vi "Kinesis - BPC301 - Connect.vi"() -> ()   [LabVIEW 2012]
uses:
  U:/Kinesis LabVIEW Website Examples/Thorlabs.MotionControl.Controls.dll
  Thorlabs.MotionControl.Controls.dll
panel:
  in  "?":bool
  in  "SerialNumber":string
  in  "BenchtopPiezoControl":refnum<k24>(container)
  # "Notes:"
  # "- Ensure that the appropriate .DLLs are copied into your Project Folder. Check that the correct bit type are used depending on your version of LabVIEW\ni.e. 32-bit or 64-bit.\n\n\n\n\n\n\n\n\n\n\n\n\n\n\n- Open the example VI through the LabVIEW Project Explorer to correctly load the User Interface from Thorlabs.MotionControl.Controls.dll."
  # "Thorlabs Hardware: BPC301 - 1-Channel Benchtop Piezo Controller\nhttps://www.thorlabs.com/newgrouppage9.cfm?objectgroup_id=1912&pn=BPC301\n\nDescription: This VI shows you how to initialize communication with and then disconnect the BPC301 controller.\n\nInstructions: \n1) Connect your BPC301 device to your PC & power the device.\nFor full device setup, the device product manual can be found on our website here. - https://www.thorlabs.com/thorproduct.cfm?partnumber=BPC301\n2) Enter the device serial number below.\n3) Click 'Run' in the LabVIEW Toolbar.\n4) To End the progam, click the 'STOP' button."
  # "Example Image of .NET Controller - VI opened via Project Explorer/ not opened via Project Explorer"
  # "VI Not Opened via Project Explorer"
  # "VI Opened via Project Explorer"
  # "- To explore the range of methods available, please visit the .NET API, included with your Kinesis software.\n\n- For tips on building your own VIs with Thorlabs Motion Control Hardware, please see our LabVIEW Guide here.\nhttps://www.thorlabs.com/newgrouppage9.cfm?objectgroup_id=10285"
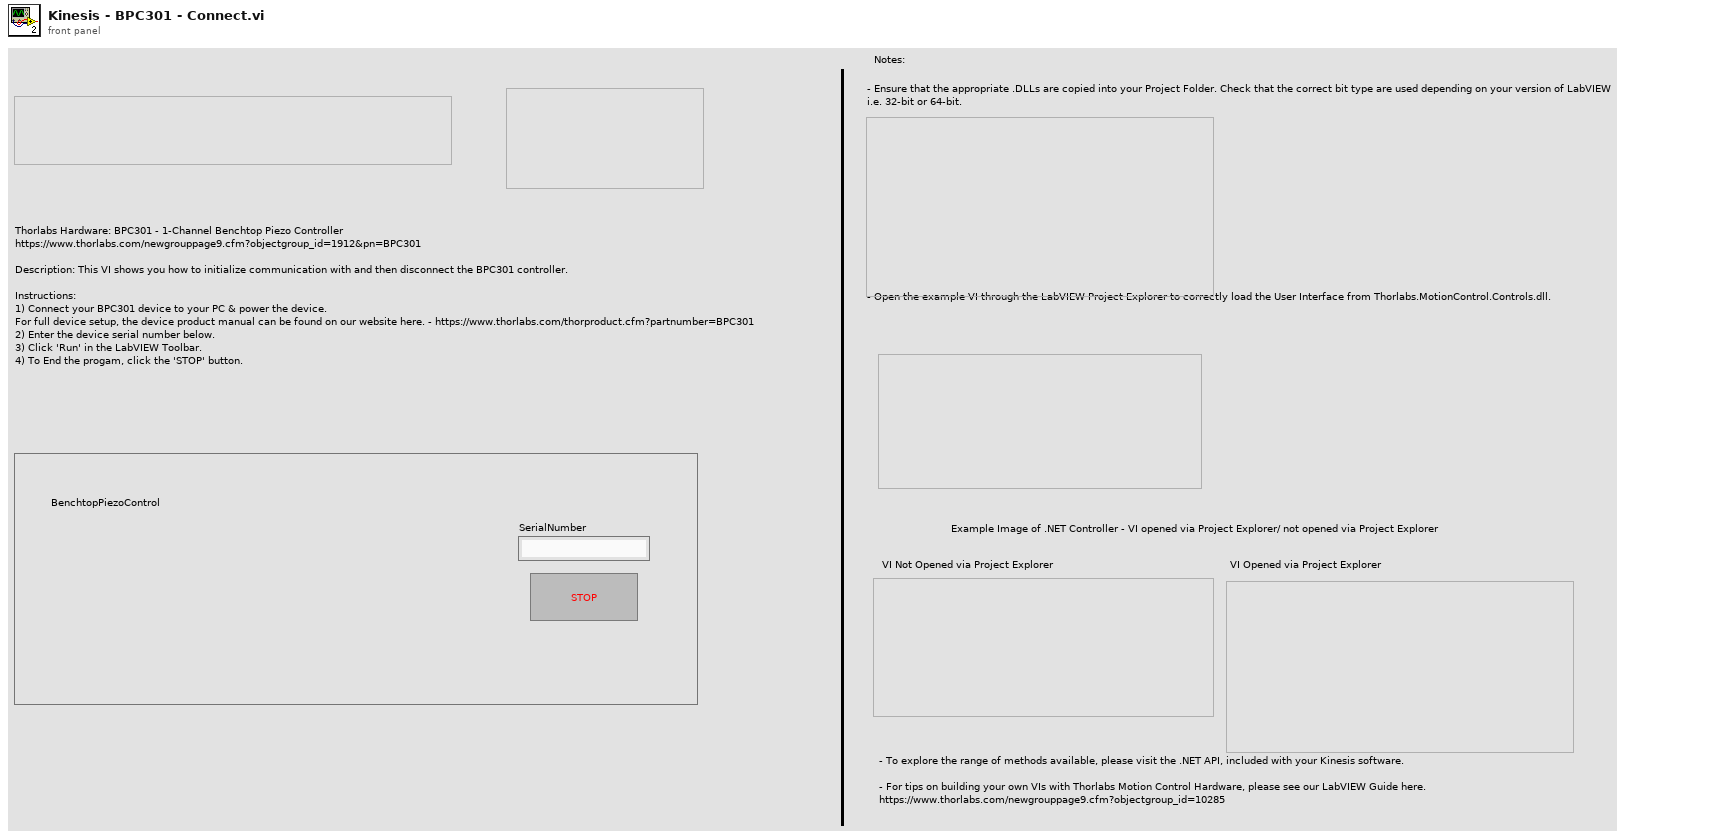
[diagram p1: front panel]
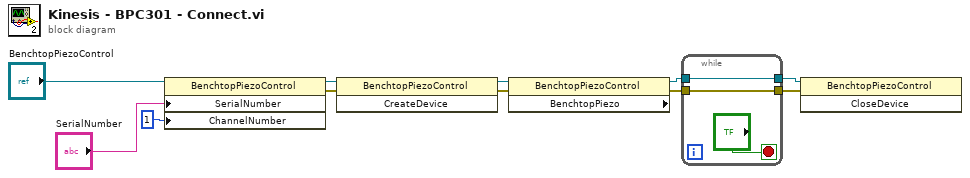
[diagram p0: block diagram]
diagram:
  n1 = property class="BenchtopPiezoControl"(reference="BenchtopPiezoControl", "SerialNumber"="SerialNumber", "ChannelNumber"=1) -> (reference out=w8:refnum<k24>, error out=w6:errorcluster)  [unwired: 1 in]
  n2 = invoke class="BenchtopPiezoControl" method="CreateDevice"(reference=w8, error in=w6) -> (reference out=w7:refnum<k24>, error out=w5:errorcluster)  [unwired: 1 in, 1 out]
  n3 = property class="BenchtopPiezoControl" props=["BenchtopPiezo"](reference=w7, error in=w5) -> (reference out=w1:refnum<k24>, error out=w3:errorcluster)  [unwired: 1 out]
  n4 = while {
    tunnel: [w14] -> w4
    tunnel: w3 -> [w14]
    tunnel: [w13] -> w2
    tunnel: w1 -> [w13]
    stop <- "?" stop-if-true
  }
  n5 = invoke class="BenchtopPiezoControl" method="CloseDevice"(reference=w2, error in=w4) -> ()  [unwired: 1 in, 3 out]
